vi "Module Name--constant.vi"(11 "Module ID":i32=-1) -> (3 "Module Name":string)   [LabVIEW 2021, in "Data Analysis.lvlib"]
doc: "Return the name of the module that owns this VI.\n_____\nBased on DQMH Project Template 6.1.0.94."
uses:
  Data Analysis.lvlib
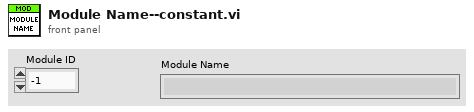
[diagram p1: front panel]
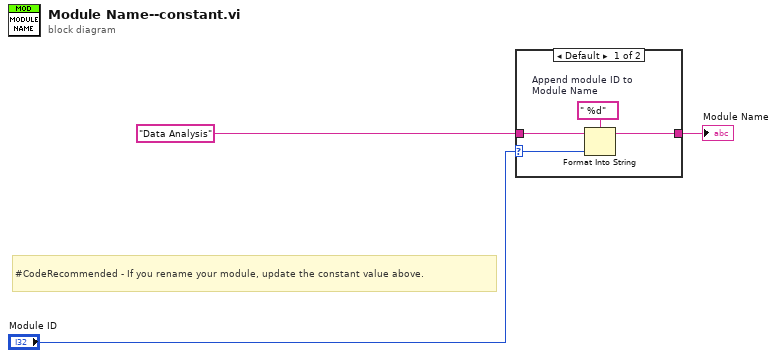
[diagram p0: block diagram]
diagram:
  # "#CodeRecommended - If you rename your module, update the constant value above."
  n1 = case shown="Default" "Module ID" {
    selector: "Module ID" -> [w5 _]
    tunnel: "Data Analysis" -> [w7 w8]
    tunnel: [w6 w8] -> w3
    frame Default {
      w4 = " %d"  # Append module ID to  Module Name
      n2 = Format Into String(format string=w4, initial string=w7, w5) -> (resulting string=w6:string)  [unwired: 1 in, 1 out]
    }
    frame ..-1 {
    }
  }
  "Module Name" <- w3
